vi "kanjam autoaim.vi"() -> ()   [LabVIEW 2013]
uses:
  Utils/Target Type.ctl
  TargetHeight.vi
  Gravity.vi
  HeightShooter.vi
panel:
  in  "Horizontal velocity":dbl
  in  "Encoder Reset":bool
  in  "Manual Fire":bool
  out "Motor Output":dbl
  in  "Target":T1 {"Orientation" format="%.2f"; "Dimensions"."Height" format="%.2f"; "Dimensions"."Width" format="%.2f"; "Center of Mass"."Y" format="%.2f"; "Center of Mass"."X" format="%.2f"; "Bounding Rect"."Bottom" format="%.2f"; "Bounding Rect"."Right" format="%.2f"; "Bounding Rect"."Top" format="%.2f"; "Bounding Rect"."Left" format="%.2f"; "Number of Holes" format="%.2f"; "Area" format="%.2f"}
  out "Rotation":dbl
  in  "Autoaim":bool
  out "Fire":bool
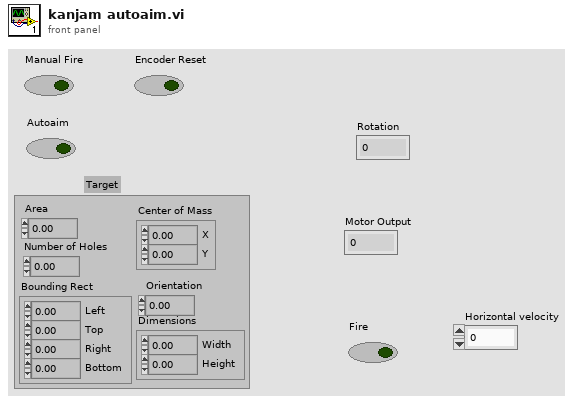
[diagram p1: front panel]
types:
  T1 = typedef "Target Type.ctl" = cluster{"Area":dbl, "Number of Holes":dbl, "Bounding Rect":cluster{"Left":dbl, "Top":dbl, "Right":dbl, "Bottom":dbl}, "Center of Mass":cluster{"X":dbl, "Y":dbl}, "Orientation":dbl, "Dimensions":cluster{"Width":dbl, "Height":dbl}}
  T2 = typedef "WPI_EncoderDevRef.ctl" = cluster{"DevStatus":errorcluster, "EncoderIndex":T3, "CounterIndex":T4, "DistancePerCount":dbl, "Decoding Type":T5}
  T3 = typedef "FPGA_EncoderIdx.ctl" = enum8{"Enc 0", "Enc 1", "Enc 2", "Enc 3", "Invalid"}
  T4 = typedef "FPGA_CounterCtrSystemIndex.ctl" = enum8{"Ctr 0", "Ctr 1", "Ctr 2", "Ctr 3", "Ctr 4", "Ctr 5", "Ctr 6", "Ctr 7", "Invalid"}
  T5 = typedef "WPI_EncoderType.ctl" = enum16{"1x", "2x", "4x"}
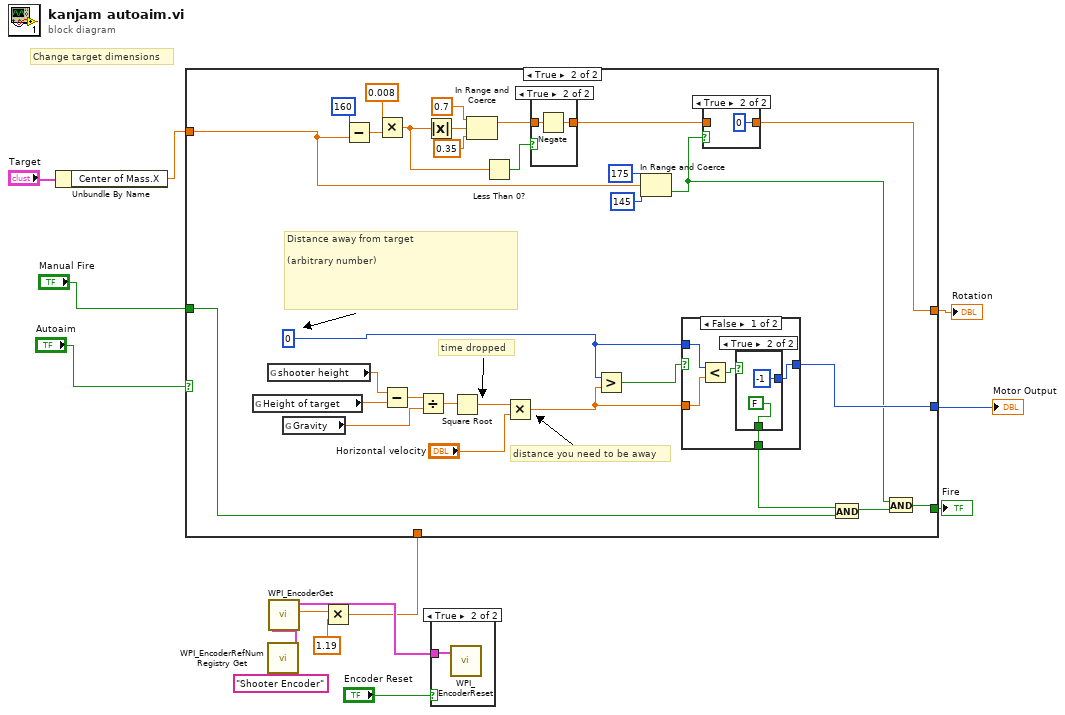
[diagram p0: block diagram]
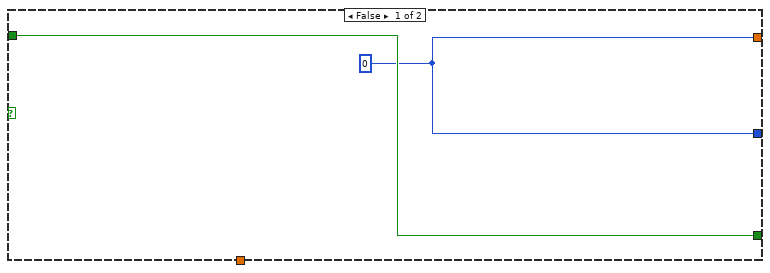
[diagram p3: hidden frame]
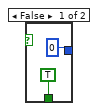
[diagram p6: hidden frame]
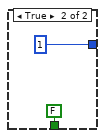
[diagram p7: hidden frame]
diagram:
  # "Change target dimensions"
  n1 = Unbundle By Name("Target") -> ("Center of Mass.X"=w1:dbl)
  n2 = call <vilib>:"WPI_EncoderRefNum Registry Get.vi"("refnum name"="Shooter Encoder") -> ("EncoderDevRef"=w8:T2)  [unwired: 9 in, 1 out]
  n3 = call <vilib>:"WPI_EncoderGet.vi"("EncoderDevRef"=w8) -> ("Distance"=w7:dbl, "EncoderDevRef"=w5:T2)  [unwired: 5 in, 4 out]
  n4 = Multiply(x=w7, y=1.19) -> (x*y=w4:dbl)
  n5 = case shown="True" "Autoaim" {
    tunnel: "Manual Fire" -> [w16 w34]
    tunnel: [w16 w19] -> w12
    tunnel: [w15 w21] -> w11
    tunnel: [w15 w38] -> w10
    tunnel: w4 -> [_ _]
    tunnel: w1 -> [_ w20]
    frame False {
      w15 = 0
    }
    frame True {
      w37 = 0
      # "distance you need to be away"
      # "time dropped"
      # "Distance away from target\n\n(arbitrary number)"
      n6 = global read "TargetHeight.vi" "Height of target"() -> (w41:dbl)
      n7 = global read "HeightShooter.vi" "shooter height"() -> (w42:dbl)
      n8 = global read "Gravity.vi" "Gravity"() -> (w40:dbl)
      n9 = Subtract(x=160, y=w20) -> (x-y=w31:dbl)
      n10 = Multiply(x=0.008, y=w31) -> (x*y=w25:dbl)
      n11 = Subtract(x=w42, y=w41) -> (x-y=w46:dbl)
      n12 = Divide(x=w46, y=w40) -> (x/y=w45:dbl)
      n13 = Absolute Value(x=w25) -> (abs(x)=w28:dbl)
      n14 = Square Root(x=w45) -> (sqrt(x)=w43:dbl)
      n15 = In Range and Coerce(upper limit=0.7, x=w28, lower limit=0.35) -> (coerced(x)=w26:dbl)  [unwired: 1 out]
      n16 = Less Than 0?(x=w25) -> (x < 0?=w27:bool)
      n17 = Multiply(x=w43, y="Horizontal velocity") -> (x*y=w36:dbl)
      n18 = case shown="True" w27 {
        tunnel: w26 -> [w49 w51]
        tunnel: [w49 w50] -> w22
        frame False {
        }
        frame True {
          n19 = Negate(x=w51) -> (-x=w50:dbl)
        }
      }
      n20 = Greater?(x=w37, y=w36) -> (0:w39:bool)
      n21 = In Range and Coerce(upper limit=175, x=w20, lower limit=145) -> (In Range?=w17:bool)  [unwired: 1 out]
      n22 = case shown="False" w39 {
        tunnel: [w53 1] -> w38
        tunnel: w37 -> [w55 _]
        tunnel: w36 -> [w54 _]
        tunnel: [w52 FALSE] -> w35
        frame False {
          n23 = Less?(x=w55, y=w54) -> (x < y?=w56:bool)
          n24 = case shown="True" w56 {
            tunnel: [0 -1] -> w53
            tunnel: [TRUE FALSE] -> w52
            frame False {
            }
            frame True {
            }
          }
        }
        frame True {
        }
      }
      n25 = case shown="True" w17 {
        tunnel: w22 -> [w47 _]
        tunnel: [w47 0] -> w21
        frame False {
        }
        frame True {
        }
      }
      n26 = And(x=w35, y=w34) -> (x .and. y?=w18:bool)
      n27 = And(x=w17, y=w18) -> (x .and. y?=w19:bool)
    }
  }
  "Fire" <- w12
  "Rotation" <- w11
  "Motor Output" <- w10
  n28 = case shown="True" "Encoder Reset" {
    tunnel: w5 -> [_ w63]
    frame False {
    }
    frame True {
      n29 = call <vilib>:"WPI_EncoderReset.vi"("EncoderDevRef"=w63) -> ()  [unwired: 9 in, 2 out]
    }
  }
